vi "load method in to cache.vi"(8 "error in (no error)":errorcluster, 10 "method name":string, 11 "Method Manager in":refnum<class "Method Manager.lvclass">) -> (0 "error out":errorcluster, 2 "found?":bool, 3 "Method Manager out":refnum<class "Method Manager.lvclass">)   [LabVIEW 2016, in "Method Manager.lvclass"]
uses:
  Method Manager.lvclass
  Method Manager.lvclass/Method Manager.ctl
  <vilib>/NI/JSON Support for LabVIEW/JSON Value/JSON Value.lvclass
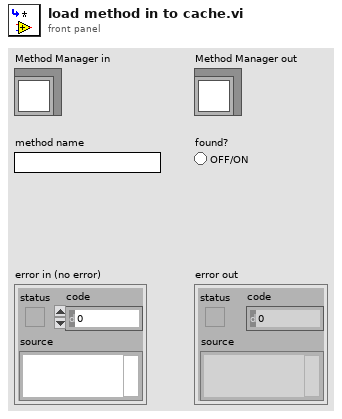
[diagram p1: front panel]
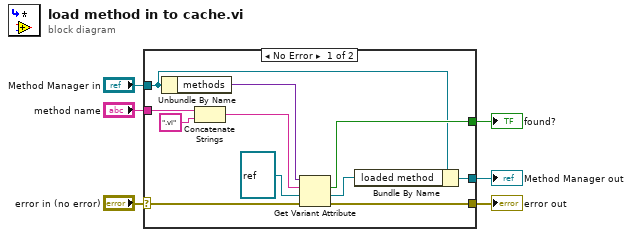
[diagram p0: block diagram]
diagram:
  n1 = case shown="No Error" "error in (no error)" {
    selector: "error in (no error)" -> [w13 w19]
    tunnel: [w16 w19] -> w3
    tunnel: [w15 _] -> w6
    tunnel: "method name" -> [w11 _]
    tunnel: "Method Manager in" -> [w7 w18]
    tunnel: [w9 w18] -> w1
    frame No Error {
      n2 = Unbundle By Name(w7) -> ("methods"=w8:variant)
      n3 = Concatenate Strings(w11, ".vi" ("string")) -> (w17:string)
      n4 = Get Variant Attribute(Variant=w8, name=w17, default value (empty Variant)=refnum<vi> refnum ("type specifier VI Refnum (for type only)"), error in=w13) -> (found=w15:bool, value=w10:refnum<vi>, error out=w16:errorcluster)  [unwired: 1 out]
      n5 = Bundle By Name(cluster=w7, "loaded method"=w10) -> (w9:refnum<class "Method Manager.lvclass">)
    }
    frame Error {
    }
  }
  "error out" <- w3
  "Method Manager out" <- w1
  "found?" <- w6
